vi "Autonomous Independent.vi"   [LabVIEW 2016]
doc: "This VI is called when autonomous begins, and will automatically be terminated when autonomous ends. You can carry out timed or sensor driven robot movement independently without needing to return to the caller."
uses:
  <vilib>/Rock Robotics/Network Tables/NT Write String.vi
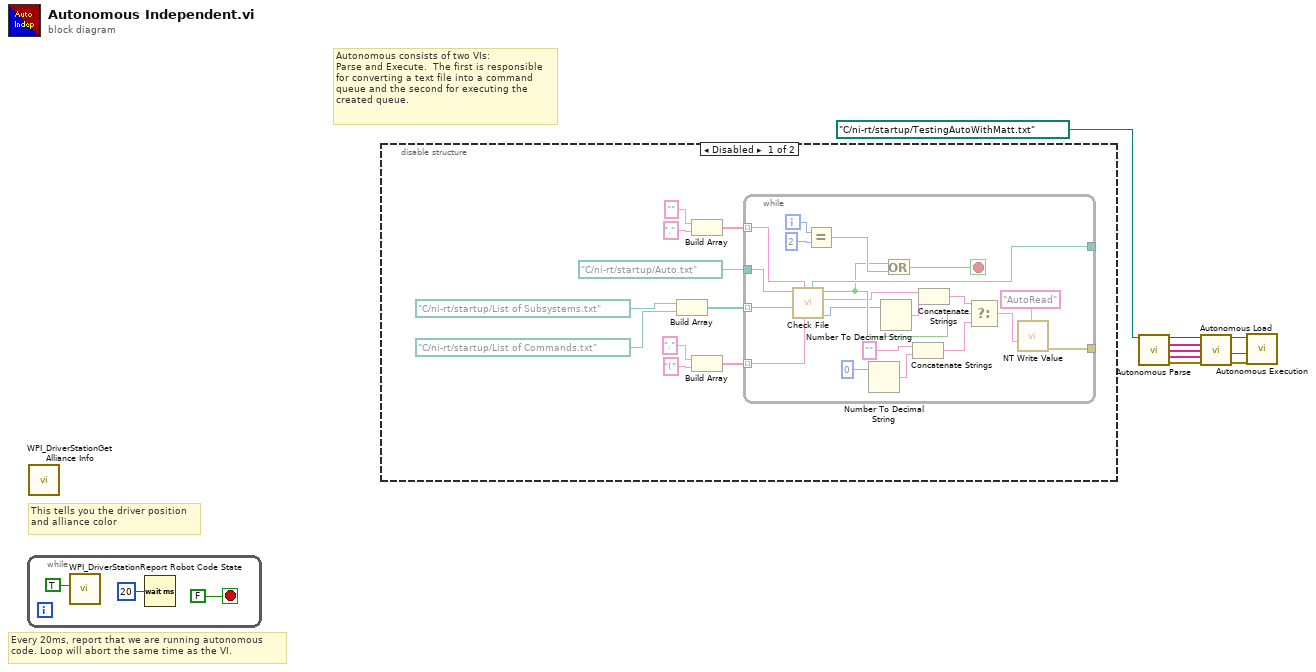
[diagram p0: block diagram]
diagram:
  # "Autonomous consists of two VIs: \nParse and Execute.  The first is responsible\nfor converting a text file into a command \nqueue and the second for executing the \ncreated queue."
  # "Every 20ms, report that we are running autonomous\ncode. Loop will abort the same time as the VI."
  # "This tells you the driver position\nand alliance color"
  n1 = while {
    stop <- FALSE stop-if-true
    n2 = call <vilib>:"WPI_DriverStationReport Robot Code State.vi"("Autonomous"=TRUE) -> ()  [unwired: 10 in, 1 out]
    n3 = Wait (ms)(milliseconds to wait=u32 20) -> ()  [unwired: 1 out]
  }
  n4 = call <vilib>:"WPI_DriverStationGet Alliance Info.vi"() -> ()  [unwired: 12 out]
  n5 = disable-structure shown="Disabled" {
    frame Disabled {
      n6 = Build Array(path "C:/ni-rt/startup/List of Subsystems.txt" ("Auto File"), path "C:/ni-rt/startup/List of Commands.txt" ("Auto File")) -> (w20:path[])
      n7 = Build Array("", ".") -> (w13:string[])
      n8 = Build Array(".", "(") -> (w18:string[])
      n9 = while {
        tunnel: path "C:/ni-rt/startup/Auto.txt" ("Auto File") -> [w43]
        tunnel: w20 -> [w42] mode=indexing
        tunnel: w18 -> [w41] mode=indexing
        tunnel: w13 -> [w40] mode=indexing
        tunnel: [w36] -> _
        tunnel: [w23] -> _
        i -> [w38]
        stop <- w35 stop-if-true
        n10 = call "Check File.vi"("Search String"=w41, "Offset String"=w40, "List of Key File"=w42, "Operative File"=w43) -> ("Line of Error"=w27:i32, "Bad String"=w26:string, "Any Errors"=w34:bool, "File Path Out"=w36:path)  [unwired: 4 in]
        n11 = Equal?(x=w38, y=2) -> (x = y?=w39:bool)
        n12 = Number To Decimal String(number=0) -> (decimal integer string=w31:string)  [unwired: 1 in]
        n13 = Number To Decimal String(number=w27) -> (decimal integer string=w29:string)  [unwired: 1 in]
        n14 = Or(x=w34, y=w39) -> (x .or. y?=w35:bool)
        n15 = Concatenate Strings("", w31) -> (w32:string)
        n16 = Concatenate Strings(w26, w29) -> (w28:string)
        n17 = Select(t=w28, s=w34, f=w32) -> (s? t:f=w25:string)
        n18 = call-poly <vilib>:"NT Write Value.vi"("String"=w25, "Name"="AutoRead") -> ("error out"=w23:errorcluster)  [unwired: 9 in]
      }
    }
    frame Enabled {
    }
  }
  n19 = call "Autonomous Parse.vi"("File Path"=path "C:/ni-rt/startup/TestingAutoWithMatt.txt" ("Auto File")) -> ("Number of Commands"=w8:i32, "Subsystems"=w7:string[], "Commands"=w6:string[], "Inputs"=w5:string[], "errror out"=w9:errorcluster)  [unwired: 8 in, 2 out]
  n20 = call "Autonomous Load.vi"("Number of Commands"=w8, "Subsystems"=w7, "Commands"=w6, "Inputs"=w5, "error in"=w9) -> ("Queue Key"=w1:refnum<queue>, "Autonomous Queue"=w2:refnum<queue>, "errror out"=w3:errorcluster)  [unwired: 8 in]
  n21 = call "Autonomous Execution.vi"("error in"=w3, "Autonomous Queue"=w2, "Queue Key"=w1) -> ()  [unwired: 9 in]
